vi "ELVIS III v1.0 Read Encoder.vi"(8 "error in (no error)":errorcluster, 9 "Reset Counter":bool, 10 "Channel":T2, 11 "myRIO Ref In":T3) -> (0 "error out":errorcluster, 1 "Counter Direction":T1, 2 "Counter Value":i32, 3 "myRIO Ref Out":T3, 5 "Overflow?":bool)   [LabVIEW 2021]
uses:
  <vilib>/myRIO/Common/Instrument Driver Framework/Utilities/typedefs/myRIO v1.0 Reference.ctl
  <vilib>/myRIO/Common/Instrument Driver Framework/Utilities/typedefs/Generic FPGA Reference.ctl
  <vilib>/myRIO/Common/Instrument Driver Framework/myRIO v1.0/Encoder/typedefs/Encoder Channels Enum.ctl
  <vilib>/myRIO/Common/Instrument Driver Framework/myRIO v1.0/Encoder/typedefs/Encoder Count Direction Enum.ctl
  <vilib>/myRIO/Common/Instrument Driver Framework/ELVIS III v1.0/Encoder/typedefs/ELVIS III Encoder Channels FPGA Reference.ctl
  <vilib>/rvi/errors/niLvFpgaAdjustHostInterfaceError.vi
  <vilib>/rvi/interface/nirviReadWriteControl/nirviReadWriteControl.xnode
  <vilib>/rvi/interface/Simulation/niFpgaSimulationCallBeginRW.vi
  NiFpgaLv.dll
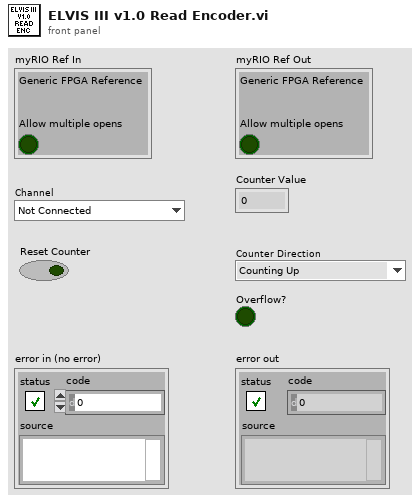
[diagram p1: front panel]
types:
  T1 = typedef "Encoder Count Direction Enum.ctl" = enum16{"Counting Up", "Counting Down"}
  T2 = typedef "Encoder Channels Enum.ctl" = enum16{"Not Connected", "C/ENC0", "C/ENC1", "A/ENC", "A/ENC0", "A/ENC1", "A/ENC2", "A/ENC3", "A/ENC4", "A/ENC5", "A/ENC6", "A/ENC7", "A/ENC8", "A/ENC9", "B/ENC", "B/ENC0", "B/ENC1", "B/ENC2", "B/ENC3", "B/ENC4", "B/ENC5", "B/ENC6", "B/ENC7", "B/ENC8", "B/ENC9", "DIO/ENC0", "DIO/ENC1", "DIO/ENC2", "DIO/ENC3", "DIO/ENC4"}
  T3 = typedef "myRIO v1.0 Reference.ctl" = cluster{"Generic FPGA Reference":T4, "Allow multiple opens":bool}
  T4 = typedef "Generic FPGA Reference.ctl" = refnum<k20>
  T5 = typedef "ELVIS III Encoder Channels FPGA Reference.ctl" = refnum<k20>
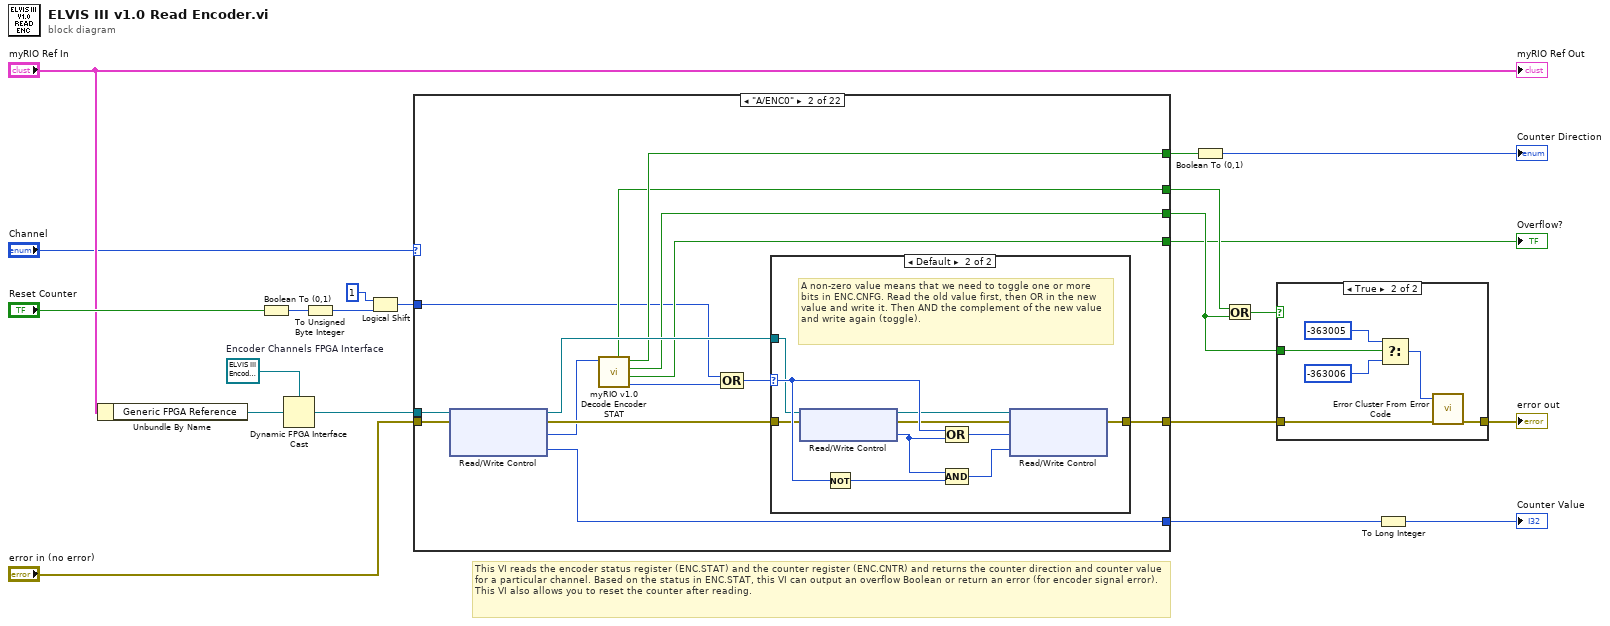
[diagram p0: block diagram]
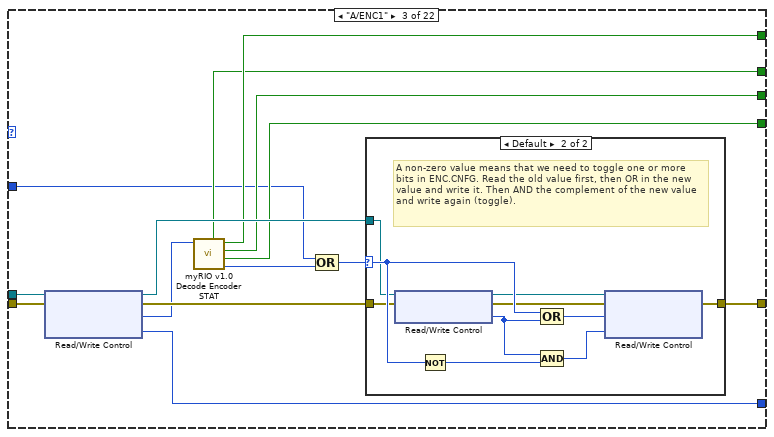
[diagram p4: hidden frame]
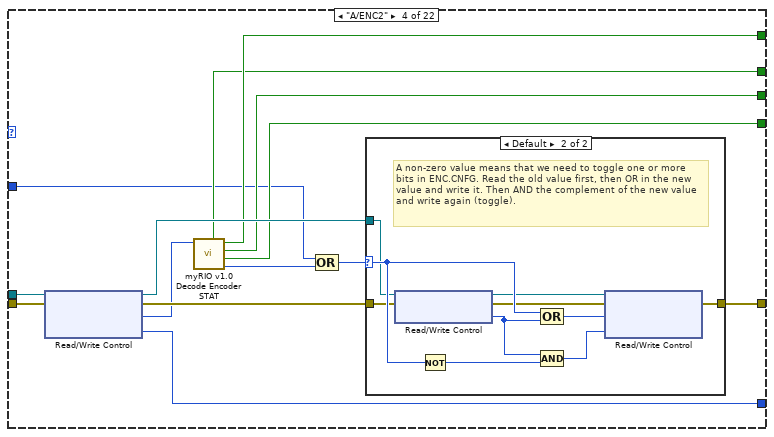
[diagram p6: hidden frame]
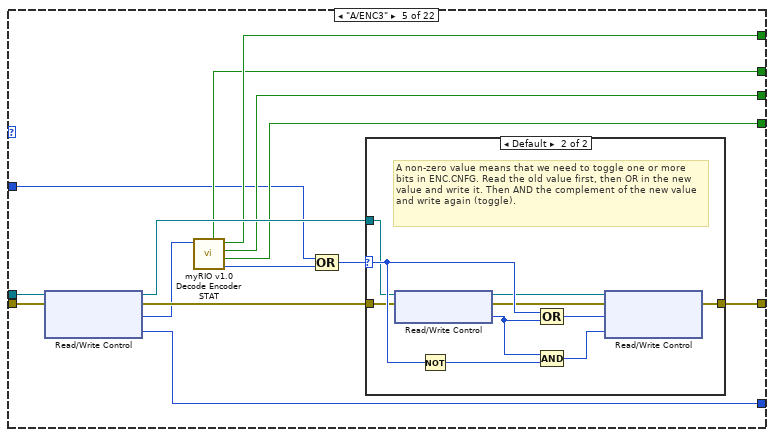
[diagram p8: hidden frame]
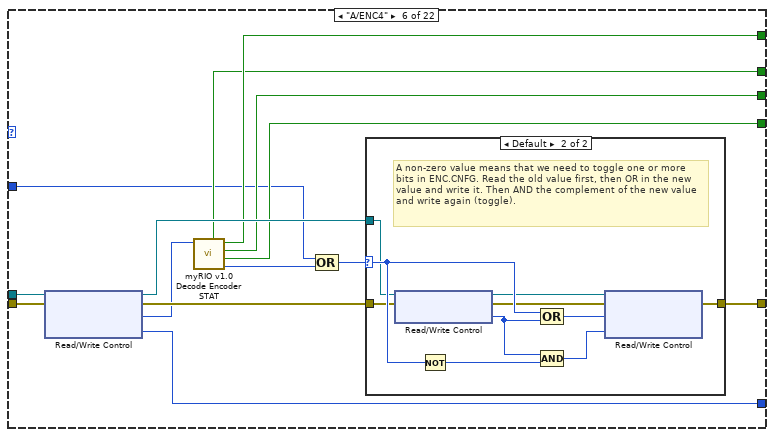
[diagram p10: hidden frame]
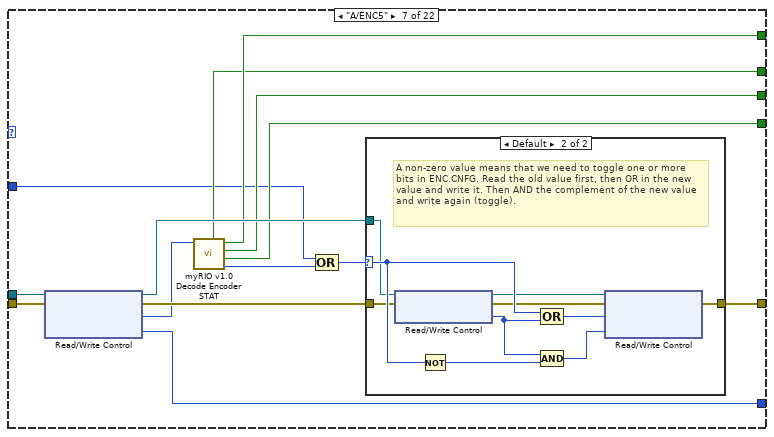
[diagram p12: hidden frame]
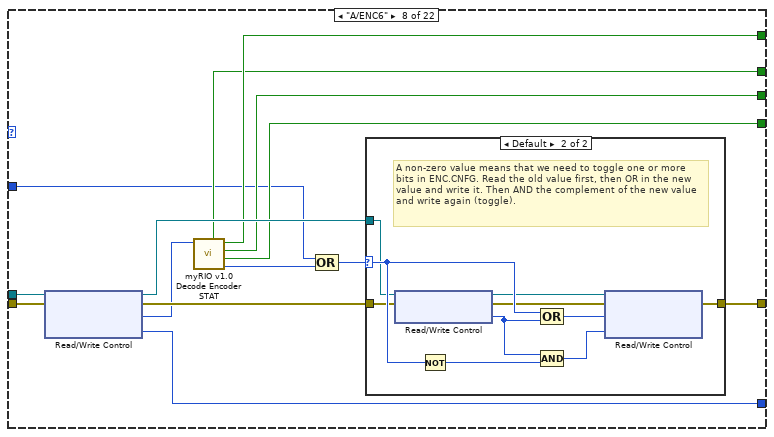
[diagram p14: hidden frame]
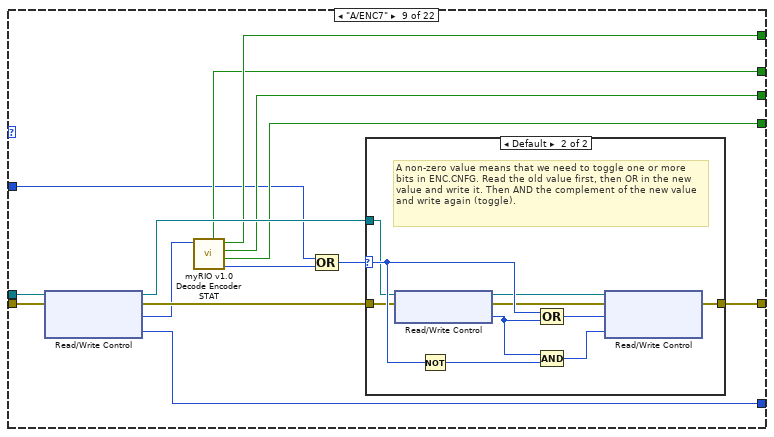
[diagram p16: hidden frame]
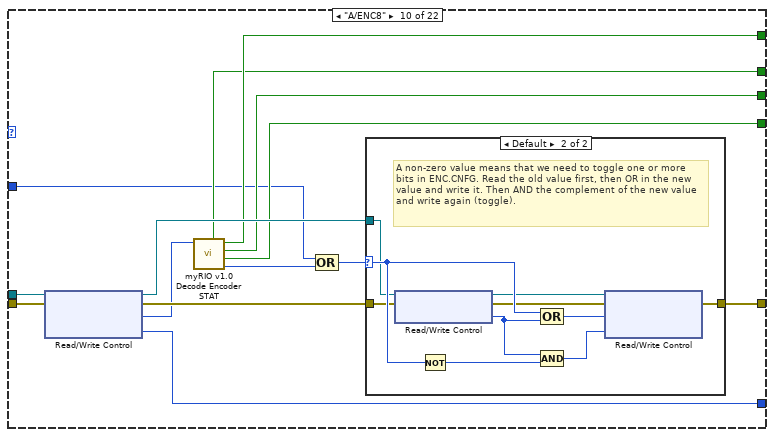
[diagram p18: hidden frame]
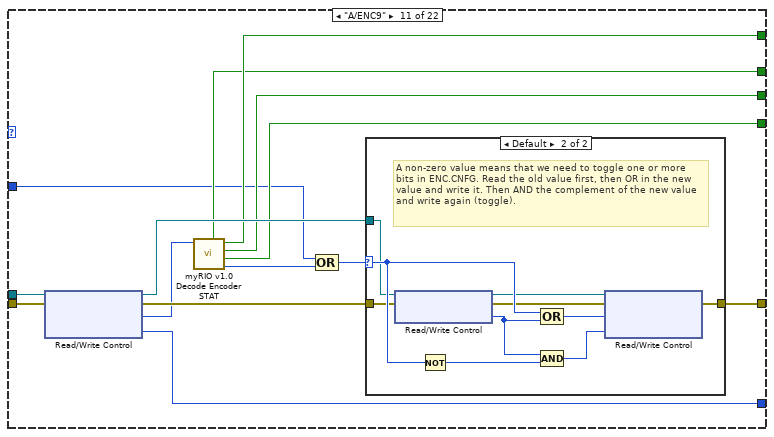
[diagram p20: hidden frame]
diagram:
  w21 = T5 refnum  # Encoder Channels FPGA Interface
  # "This VI reads the encoder status register (ENC.STAT) and the counter register (ENC.CNTR) and returns the counter direction and counter value for a particular channel. Based on the status in ENC.STAT, this VI can output an overflow Boolean or return an error (for encoder signal error). This VI also allows you to reset the counter after reading."
  n1 = Unbundle By Name("myRIO Ref In") -> ("Generic FPGA Reference"=w14:T4)
  n2 = Boolean To (0,1)(Boolean="Reset Counter") -> (0, 1=w15:i16)
  n3 = Dynamic FPGA Interface Cast(Session In=w21, Type=w14) -> (Session Out=w1:T5)
  n4 = To Unsigned Byte Integer(number=w15) -> (unsigned 8bit integer=w16:u8)
  n5 = Logical Shift(y=u8 1, x=w16) -> (x << y=w2:u8)
  n6 = case shown="\"A/ENC0\"" "Channel" {
    tunnel: "error in (no error)" -> [w22 w30 w55 w80 w105 w130 w155 w180 w205 w230 w255 w280 w305 w330 w355 w380 w405 w430 w455 w480 w505 w526]
    tunnel: [w22 w25 w50 w75 w100 w125 w150 w175 w200 w225 w250 w275 w300 w325 w350 w375 w400 w425 w450 w475 w500 w525] -> w9
    tunnel: [_ w24 w49 w74 w99 w124 w149 w174 w199 w224 w249 w274 w299 w324 w349 w374 w399 w424 w449 w474 w499 w524] -> w8
    tunnel: [_ w29 w54 w79 w104 w129 w154 w179 w204 w229 w254 w279 w304 w329 w354 w379 w404 w429 w454 w479 w504 w523] -> w7
    tunnel: [_ w28 w53 w78 w103 w128 w153 w178 w203 w228 w253 w278 w303 w328 w353 w378 w403 w428 w453 w478 w503 w523] -> w6
    tunnel: [_ w27 w52 w77 w102 w127 w152 w177 w202 w227 w252 w277 w302 w327 w352 w377 w402 w427 w452 w477 w502 w523] -> w5
    tunnel: [_ w26 w51 w76 w101 w126 w151 w176 w201 w226 w251 w276 w301 w326 w351 w376 w401 w426 w451 w476 w501 w523] -> w4
    tunnel: w2 -> [_ w23 w48 w73 w98 w123 w148 w173 w198 w223 w248 w273 w298 w323 w348 w373 w398 w423 w448 w473 w498 _]
    tunnel: w1 -> [_ w31 w56 w81 w106 w131 w156 w181 w206 w231 w256 w281 w306 w331 w356 w381 w406 w431 w456 w481 w506 _]
    frame "Not Connected" {
    }
    frame "A/ENC0" {
      n7 = xnode "Read/Write Control"("FPGA VI Reference In"=w31, "error in"=w30) -> ("FPGA VI Reference Out"=w34:T5, "error out"=w33:errorcluster, "ENC.A_0.STAT"=w32:u8, "ENC.A_0.CNTR"=w24:u32)
      n8 = call <vilib>:"myRIO v1.0 Decode Encoder STAT.vi"("ENC.STAT"=w32) -> ("ENC.CNFG to write"=w35:u8, "Signed Overflow?"=w26:bool, "Error?"=w27:bool, "Counting down?"=w29:bool, "Signed Overflow Error?"=w28:bool)  [unwired: 6 in]
      n9 = Compound Arithmetic op=OR(w23, w35) -> (w36:u8)
      n10 = case shown="Default" w36 {
        selector: w36 -> [_ w46]
        tunnel: w34 -> [_ w45]
        tunnel: w33 -> [w37 w44]
        tunnel: [w37 w38] -> w25
        frame 0 {
        }
        frame Default {
          # "A non-zero value means that we need to toggle one or more bits in ENC.CNFG. Read the old value first, then OR in the new value and write it. Then AND the complement of the new value and write again (toggle)."
          n11 = xnode "Read/Write Control"("FPGA VI Reference In"=w45, "error in"=w44) -> ("FPGA VI Reference Out"=w42:T5, "error out"=w41:errorcluster, "ENC.A_0.CNFG"=w43:u8)
          n12 = Not(x=w46) -> (.not. x?=w47:u8)
          n13 = Compound Arithmetic op=OR(w46, w43) -> (w40:u8)
          n14 = Compound Arithmetic op=AND(w43, w47) -> (w39:u8)
          n15 = xnode "Read/Write Control"("FPGA VI Reference In"=w42, "error in"=w41, "ENC.A_0.CNFG"=w40, "ENC.A_0.CNFG"=w39) -> ("error out"=w38:errorcluster)  [unwired: 1 out]
        }
      }
    }
    frame "A/ENC1" {
      n16 = xnode "Read/Write Control"("FPGA VI Reference In"=w56, "error in"=w55) -> ("FPGA VI Reference Out"=w59:T5, "error out"=w58:errorcluster, "ENC.A_1.STAT"=w57:u8, "ENC.A_1.CNTR"=w49:u32)
      n17 = call <vilib>:"myRIO v1.0 Decode Encoder STAT.vi"("ENC.STAT"=w57) -> ("ENC.CNFG to write"=w60:u8, "Signed Overflow?"=w51:bool, "Error?"=w52:bool, "Counting down?"=w54:bool, "Signed Overflow Error?"=w53:bool)  [unwired: 6 in]
      n18 = Compound Arithmetic op=OR(w48, w60) -> (w61:u8)
      n19 = case shown="Default" w61 {
        selector: w61 -> [_ w71]
        tunnel: w59 -> [_ w70]
        tunnel: w58 -> [w62 w69]
        tunnel: [w62 w63] -> w50
        frame 0 {
        }
        frame Default {
          # "A non-zero value means that we need to toggle one or more bits in ENC.CNFG. Read the old value first, then OR in the new value and write it. Then AND the complement of the new value and write again (toggle)."
          n20 = xnode "Read/Write Control"("FPGA VI Reference In"=w70, "error in"=w69) -> ("FPGA VI Reference Out"=w67:T5, "error out"=w66:errorcluster, "ENC.A_1.CNFG"=w68:u8)
          n21 = Not(x=w71) -> (.not. x?=w72:u8)
          n22 = Compound Arithmetic op=OR(w71, w68) -> (w65:u8)
          n23 = Compound Arithmetic op=AND(w68, w72) -> (w64:u8)
          n24 = xnode "Read/Write Control"("FPGA VI Reference In"=w67, "error in"=w66, "ENC.A_1.CNFG"=w65, "ENC.A_1.CNFG"=w64) -> ("error out"=w63:errorcluster)  [unwired: 1 out]
        }
      }
    }
    frame "A/ENC2" {
      n25 = xnode "Read/Write Control"("FPGA VI Reference In"=w81, "error in"=w80) -> ("FPGA VI Reference Out"=w84:T5, "error out"=w83:errorcluster, "ENC.A_2.STAT"=w82:u8, "ENC.A_2.CNTR"=w74:u32)
      n26 = call <vilib>:"myRIO v1.0 Decode Encoder STAT.vi"("ENC.STAT"=w82) -> ("ENC.CNFG to write"=w85:u8, "Signed Overflow?"=w76:bool, "Error?"=w77:bool, "Counting down?"=w79:bool, "Signed Overflow Error?"=w78:bool)  [unwired: 6 in]
      n27 = Compound Arithmetic op=OR(w73, w85) -> (w86:u8)
      n28 = case shown="Default" w86 {
        selector: w86 -> [_ w96]
        tunnel: w84 -> [_ w95]
        tunnel: w83 -> [w87 w94]
        tunnel: [w87 w88] -> w75
        frame 0 {
        }
        frame Default {
          # "A non-zero value means that we need to toggle one or more bits in ENC.CNFG. Read the old value first, then OR in the new value and write it. Then AND the complement of the new value and write again (toggle)."
          n29 = xnode "Read/Write Control"("FPGA VI Reference In"=w95, "error in"=w94) -> ("FPGA VI Reference Out"=w92:T5, "error out"=w91:errorcluster, "ENC.A_2.CNFG"=w93:u8)
          n30 = Not(x=w96) -> (.not. x?=w97:u8)
          n31 = Compound Arithmetic op=OR(w96, w93) -> (w90:u8)
          n32 = Compound Arithmetic op=AND(w93, w97) -> (w89:u8)
          n33 = xnode "Read/Write Control"("FPGA VI Reference In"=w92, "error in"=w91, "ENC.A_2.CNFG"=w90, "ENC.A_2.CNFG"=w89) -> ("error out"=w88:errorcluster)  [unwired: 1 out]
        }
      }
    }
    frame "A/ENC3" {
      n34 = xnode "Read/Write Control"("FPGA VI Reference In"=w106, "error in"=w105) -> ("FPGA VI Reference Out"=w109:T5, "error out"=w108:errorcluster, "ENC.A_3.STAT"=w107:u8, "ENC.A_3.CNTR"=w99:u32)
      n35 = call <vilib>:"myRIO v1.0 Decode Encoder STAT.vi"("ENC.STAT"=w107) -> ("ENC.CNFG to write"=w110:u8, "Signed Overflow?"=w101:bool, "Error?"=w102:bool, "Counting down?"=w104:bool, "Signed Overflow Error?"=w103:bool)  [unwired: 6 in]
      n36 = Compound Arithmetic op=OR(w98, w110) -> (w111:u8)
      n37 = case shown="Default" w111 {
        selector: w111 -> [_ w121]
        tunnel: w109 -> [_ w120]
        tunnel: w108 -> [w112 w119]
        tunnel: [w112 w113] -> w100
        frame 0 {
        }
        frame Default {
          # "A non-zero value means that we need to toggle one or more bits in ENC.CNFG. Read the old value first, then OR in the new value and write it. Then AND the complement of the new value and write again (toggle)."
          n38 = xnode "Read/Write Control"("FPGA VI Reference In"=w120, "error in"=w119) -> ("FPGA VI Reference Out"=w117:T5, "error out"=w116:errorcluster, "ENC.A_3.CNFG"=w118:u8)
          n39 = Not(x=w121) -> (.not. x?=w122:u8)
          n40 = Compound Arithmetic op=OR(w121, w118) -> (w115:u8)
          n41 = Compound Arithmetic op=AND(w118, w122) -> (w114:u8)
          n42 = xnode "Read/Write Control"("FPGA VI Reference In"=w117, "error in"=w116, "ENC.A_3.CNFG"=w115, "ENC.A_3.CNFG"=w114) -> ("error out"=w113:errorcluster)  [unwired: 1 out]
        }
      }
    }
    frame "A/ENC4" {
      n43 = xnode "Read/Write Control"("FPGA VI Reference In"=w131, "error in"=w130) -> ("FPGA VI Reference Out"=w134:T5, "error out"=w133:errorcluster, "ENC.A_4.STAT"=w132:u8, "ENC.A_4.CNTR"=w124:u32)
      n44 = call <vilib>:"myRIO v1.0 Decode Encoder STAT.vi"("ENC.STAT"=w132) -> ("ENC.CNFG to write"=w135:u8, "Signed Overflow?"=w126:bool, "Error?"=w127:bool, "Counting down?"=w129:bool, "Signed Overflow Error?"=w128:bool)  [unwired: 6 in]
      n45 = Compound Arithmetic op=OR(w123, w135) -> (w136:u8)
      n46 = case shown="Default" w136 {
        selector: w136 -> [_ w146]
        tunnel: w134 -> [_ w145]
        tunnel: w133 -> [w137 w144]
        tunnel: [w137 w138] -> w125
        frame 0 {
        }
        frame Default {
          # "A non-zero value means that we need to toggle one or more bits in ENC.CNFG. Read the old value first, then OR in the new value and write it. Then AND the complement of the new value and write again (toggle)."
          n47 = xnode "Read/Write Control"("FPGA VI Reference In"=w145, "error in"=w144) -> ("FPGA VI Reference Out"=w142:T5, "error out"=w141:errorcluster, "ENC.A_4.CNFG"=w143:u8)
          n48 = Not(x=w146) -> (.not. x?=w147:u8)
          n49 = Compound Arithmetic op=OR(w146, w143) -> (w140:u8)
          n50 = Compound Arithmetic op=AND(w143, w147) -> (w139:u8)
          n51 = xnode "Read/Write Control"("FPGA VI Reference In"=w142, "error in"=w141, "ENC.A_4.CNFG"=w140, "ENC.A_4.CNFG"=w139) -> ("error out"=w138:errorcluster)  [unwired: 1 out]
        }
      }
    }
    frame "A/ENC5" {
      n52 = xnode "Read/Write Control"("FPGA VI Reference In"=w156, "error in"=w155) -> ("FPGA VI Reference Out"=w159:T5, "error out"=w158:errorcluster, "ENC.A_5.STAT"=w157:u8, "ENC.A_5.CNTR"=w149:u32)
      n53 = call <vilib>:"myRIO v1.0 Decode Encoder STAT.vi"("ENC.STAT"=w157) -> ("ENC.CNFG to write"=w160:u8, "Signed Overflow?"=w151:bool, "Error?"=w152:bool, "Counting down?"=w154:bool, "Signed Overflow Error?"=w153:bool)  [unwired: 6 in]
      n54 = Compound Arithmetic op=OR(w148, w160) -> (w161:u8)
      n55 = case shown="Default" w161 {
        selector: w161 -> [_ w171]
        tunnel: w159 -> [_ w170]
        tunnel: w158 -> [w162 w169]
        tunnel: [w162 w163] -> w150
        frame 0 {
        }
        frame Default {
          # "A non-zero value means that we need to toggle one or more bits in ENC.CNFG. Read the old value first, then OR in the new value and write it. Then AND the complement of the new value and write again (toggle)."
          n56 = xnode "Read/Write Control"("FPGA VI Reference In"=w170, "error in"=w169) -> ("FPGA VI Reference Out"=w167:T5, "error out"=w166:errorcluster, "ENC.A_5.CNFG"=w168:u8)
          n57 = Not(x=w171) -> (.not. x?=w172:u8)
          n58 = Compound Arithmetic op=OR(w171, w168) -> (w165:u8)
          n59 = Compound Arithmetic op=AND(w168, w172) -> (w164:u8)
          n60 = xnode "Read/Write Control"("FPGA VI Reference In"=w167, "error in"=w166, "ENC.A_5.CNFG"=w165, "ENC.A_5.CNFG"=w164) -> ("error out"=w163:errorcluster)  [unwired: 1 out]
        }
      }
    }
    frame "A/ENC6" {
      n61 = xnode "Read/Write Control"("FPGA VI Reference In"=w181, "error in"=w180) -> ("FPGA VI Reference Out"=w184:T5, "error out"=w183:errorcluster, "ENC.A_6.STAT"=w182:u8, "ENC.A_6.CNTR"=w174:u32)
      n62 = call <vilib>:"myRIO v1.0 Decode Encoder STAT.vi"("ENC.STAT"=w182) -> ("ENC.CNFG to write"=w185:u8, "Signed Overflow?"=w176:bool, "Error?"=w177:bool, "Counting down?"=w179:bool, "Signed Overflow Error?"=w178:bool)  [unwired: 6 in]
      n63 = Compound Arithmetic op=OR(w173, w185) -> (w186:u8)
      n64 = case shown="Default" w186 {
        selector: w186 -> [_ w196]
        tunnel: w184 -> [_ w195]
        tunnel: w183 -> [w187 w194]
        tunnel: [w187 w188] -> w175
        frame 0 {
        }
        frame Default {
          # "A non-zero value means that we need to toggle one or more bits in ENC.CNFG. Read the old value first, then OR in the new value and write it. Then AND the complement of the new value and write again (toggle)."
          n65 = xnode "Read/Write Control"("FPGA VI Reference In"=w195, "error in"=w194) -> ("FPGA VI Reference Out"=w192:T5, "error out"=w191:errorcluster, "ENC.A_6.CNFG"=w193:u8)
          n66 = Not(x=w196) -> (.not. x?=w197:u8)
          n67 = Compound Arithmetic op=OR(w196, w193) -> (w190:u8)
          n68 = Compound Arithmetic op=AND(w193, w197) -> (w189:u8)
          n69 = xnode "Read/Write Control"("FPGA VI Reference In"=w192, "error in"=w191, "ENC.A_6.CNFG"=w190, "ENC.A_6.CNFG"=w189) -> ("error out"=w188:errorcluster)  [unwired: 1 out]
        }
      }
    }
    frame "A/ENC7" {
      n70 = xnode "Read/Write Control"("FPGA VI Reference In"=w206, "error in"=w205) -> ("FPGA VI Reference Out"=w209:T5, "error out"=w208:errorcluster, "ENC.A_7.STAT"=w207:u8, "ENC.A_7.CNTR"=w199:u32)
      n71 = call <vilib>:"myRIO v1.0 Decode Encoder STAT.vi"("ENC.STAT"=w207) -> ("ENC.CNFG to write"=w210:u8, "Signed Overflow?"=w201:bool, "Error?"=w202:bool, "Counting down?"=w204:bool, "Signed Overflow Error?"=w203:bool)  [unwired: 6 in]
      n72 = Compound Arithmetic op=OR(w198, w210) -> (w211:u8)
      n73 = case shown="Default" w211 {
        selector: w211 -> [_ w221]
        tunnel: w209 -> [_ w220]
        tunnel: w208 -> [w212 w219]
        tunnel: [w212 w213] -> w200
        frame 0 {
        }
        frame Default {
          # "A non-zero value means that we need to toggle one or more bits in ENC.CNFG. Read the old value first, then OR in the new value and write it. Then AND the complement of the new value and write again (toggle)."
          n74 = xnode "Read/Write Control"("FPGA VI Reference In"=w220, "error in"=w219) -> ("FPGA VI Reference Out"=w217:T5, "error out"=w216:errorcluster, "ENC.A_7.CNFG"=w218:u8)
          n75 = Not(x=w221) -> (.not. x?=w222:u8)
          n76 = Compound Arithmetic op=OR(w221, w218) -> (w215:u8)
          n77 = Compound Arithmetic op=AND(w218, w222) -> (w214:u8)
          n78 = xnode "Read/Write Control"("FPGA VI Reference In"=w217, "error in"=w216, "ENC.A_7.CNFG"=w215, "ENC.A_7.CNFG"=w214) -> ("error out"=w213:errorcluster)  [unwired: 1 out]
        }
      }
    }
    frame "A/ENC8" {
      n79 = xnode "Read/Write Control"("FPGA VI Reference In"=w231, "error in"=w230) -> ("FPGA VI Reference Out"=w234:T5, "error out"=w233:errorcluster, "ENC.A_8.STAT"=w232:u8, "ENC.A_8.CNTR"=w224:u32)
      n80 = call <vilib>:"myRIO v1.0 Decode Encoder STAT.vi"("ENC.STAT"=w232) -> ("ENC.CNFG to write"=w235:u8, "Signed Overflow?"=w226:bool, "Error?"=w227:bool, "Counting down?"=w229:bool, "Signed Overflow Error?"=w228:bool)  [unwired: 6 in]
      n81 = Compound Arithmetic op=OR(w223, w235) -> (w236:u8)
      n82 = case shown="Default" w236 {
        selector: w236 -> [_ w246]
        tunnel: w234 -> [_ w245]
        tunnel: w233 -> [w237 w244]
        tunnel: [w237 w238] -> w225
        frame 0 {
        }
        frame Default {
          # "A non-zero value means that we need to toggle one or more bits in ENC.CNFG. Read the old value first, then OR in the new value and write it. Then AND the complement of the new value and write again (toggle)."
          n83 = xnode "Read/Write Control"("FPGA VI Reference In"=w245, "error in"=w244) -> ("FPGA VI Reference Out"=w242:T5, "error out"=w241:errorcluster, "ENC.A_8.CNFG"=w243:u8)
          n84 = Not(x=w246) -> (.not. x?=w247:u8)
          n85 = Compound Arithmetic op=OR(w246, w243) -> (w240:u8)
          n86 = Compound Arithmetic op=AND(w243, w247) -> (w239:u8)
          n87 = xnode "Read/Write Control"("FPGA VI Reference In"=w242, "error in"=w241, "ENC.A_8.CNFG"=w240, "ENC.A_8.CNFG"=w239) -> ("error out"=w238:errorcluster)  [unwired: 1 out]
        }
      }
    }
    frame "A/ENC9" {
      n88 = xnode "Read/Write Control"("FPGA VI Reference In"=w256, "error in"=w255) -> ("FPGA VI Reference Out"=w259:T5, "error out"=w258:errorcluster, "ENC.A_9.STAT"=w257:u8, "ENC.A_9.CNTR"=w249:u32)
      n89 = call <vilib>:"myRIO v1.0 Decode Encoder STAT.vi"("ENC.STAT"=w257) -> ("ENC.CNFG to write"=w260:u8, "Signed Overflow?"=w251:bool, "Error?"=w252:bool, "Counting down?"=w254:bool, "Signed Overflow Error?"=w253:bool)  [unwired: 6 in]
      n90 = Compound Arithmetic op=OR(w248, w260) -> (w261:u8)
      n91 = case shown="Default" w261 {
        selector: w261 -> [_ w271]
        tunnel: w259 -> [_ w270]
        tunnel: w258 -> [w262 w269]
        tunnel: [w262 w263] -> w250
        frame 0 {
        }
        frame Default {
          # "A non-zero value means that we need to toggle one or more bits in ENC.CNFG. Read the old value first, then OR in the new value and write it. Then AND the complement of the new value and write again (toggle)."
          n92 = xnode "Read/Write Control"("FPGA VI Reference In"=w270, "error in"=w269) -> ("FPGA VI Reference Out"=w267:T5, "error out"=w266:errorcluster, "ENC.A_9.CNFG"=w268:u8)
          n93 = Not(x=w271) -> (.not. x?=w272:u8)
          n94 = Compound Arithmetic op=OR(w271, w268) -> (w265:u8)
          n95 = Compound Arithmetic op=AND(w268, w272) -> (w264:u8)
          n96 = xnode "Read/Write Control"("FPGA VI Reference In"=w267, "error in"=w266, "ENC.A_9.CNFG"=w265, "ENC.A_9.CNFG"=w264) -> ("error out"=w263:errorcluster)  [unwired: 1 out]
        }
      }
    }
    frame "B/ENC0" {
      n97 = xnode "Read/Write Control"("FPGA VI Reference In"=w281, "error in"=w280) -> ("FPGA VI Reference Out"=w284:T5, "error out"=w283:errorcluster, "ENC.B_0.STAT"=w282:u8, "ENC.B_0.CNTR"=w274:u32)
      n98 = call <vilib>:"myRIO v1.0 Decode Encoder STAT.vi"("ENC.STAT"=w282) -> ("ENC.CNFG to write"=w285:u8, "Signed Overflow?"=w276:bool, "Error?"=w277:bool, "Counting down?"=w279:bool, "Signed Overflow Error?"=w278:bool)  [unwired: 6 in]
      n99 = Compound Arithmetic op=OR(w273, w285) -> (w286:u8)
      n100 = case shown="Default" w286 {
        selector: w286 -> [_ w296]
        tunnel: w284 -> [_ w295]
        tunnel: w283 -> [w287 w294]
        tunnel: [w287 w288] -> w275
        frame 0 {
        }
        frame Default {
          # "A non-zero value means that we need to toggle one or more bits in ENC.CNFG. Read the old value first, then OR in the new value and write it. Then AND the complement of the new value and write again (toggle)."
          n101 = xnode "Read/Write Control"("FPGA VI Reference In"=w295, "error in"=w294) -> ("FPGA VI Reference Out"=w292:T5, "error out"=w291:errorcluster, "ENC.B_0.CNFG"=w293:u8)
          n102 = Not(x=w296) -> (.not. x?=w297:u8)
          n103 = Compound Arithmetic op=OR(w296, w293) -> (w290:u8)
          n104 = Compound Arithmetic op=AND(w293, w297) -> (w289:u8)
          n105 = xnode "Read/Write Control"("FPGA VI Reference In"=w292, "error in"=w291, "ENC.B_0.CNFG"=w290, "ENC.B_0.CNFG"=w289) -> ("error out"=w288:errorcluster)  [unwired: 1 out]
        }
      }
    }
    frame "B/ENC1" {
      n106 = xnode "Read/Write Control"("FPGA VI Reference In"=w306, "error in"=w305) -> ("FPGA VI Reference Out"=w309:T5, "error out"=w308:errorcluster, "ENC.B_1.STAT"=w307:u8, "ENC.B_1.CNTR"=w299:u32)
      n107 = call <vilib>:"myRIO v1.0 Decode Encoder STAT.vi"("ENC.STAT"=w307) -> ("ENC.CNFG to write"=w310:u8, "Signed Overflow?"=w301:bool, "Error?"=w302:bool, "Counting down?"=w304:bool, "Signed Overflow Error?"=w303:bool)  [unwired: 6 in]
      n108 = Compound Arithmetic op=OR(w298, w310) -> (w311:u8)
      n109 = case shown="Default" w311 {
        selector: w311 -> [_ w321]
        tunnel: w309 -> [_ w320]
        tunnel: w308 -> [w312 w319]
        tunnel: [w312 w313] -> w300
        frame 0 {
        }
        frame Default {
          # "A non-zero value means that we need to toggle one or more bits in ENC.CNFG. Read the old value first, then OR in the new value and write it. Then AND the complement of the new value and write again (toggle)."
          n110 = xnode "Read/Write Control"("FPGA VI Reference In"=w320, "error in"=w319) -> ("FPGA VI Reference Out"=w317:T5, "error out"=w316:errorcluster, "ENC.B_1.CNFG"=w318:u8)
          n111 = Not(x=w321) -> (.not. x?=w322:u8)
          n112 = Compound Arithmetic op=OR(w321, w318) -> (w315:u8)
          n113 = Compound Arithmetic op=AND(w318, w322) -> (w314:u8)
          n114 = xnode "Read/Write Control"("FPGA VI Reference In"=w317, "error in"=w316, "ENC.B_1.CNFG"=w315, "ENC.B_1.CNFG"=w314) -> ("error out"=w313:errorcluster)  [unwired: 1 out]
        }
      }
    }
    frame "B/ENC2" {
      n115 = xnode "Read/Write Control"("FPGA VI Reference In"=w331, "error in"=w330) -> ("FPGA VI Reference Out"=w334:T5, "error out"=w333:errorcluster, "ENC.B_2.STAT"=w332:u8, "ENC.B_2.CNTR"=w324:u32)
      n116 = call <vilib>:"myRIO v1.0 Decode Encoder STAT.vi"("ENC.STAT"=w332) -> ("ENC.CNFG to write"=w335:u8, "Signed Overflow?"=w326:bool, "Error?"=w327:bool, "Counting down?"=w329:bool, "Signed Overflow Error?"=w328:bool)  [unwired: 6 in]
      n117 = Compound Arithmetic op=OR(w323, w335) -> (w336:u8)
      n118 = case shown="Default" w336 {
        selector: w336 -> [_ w346]
        tunnel: w334 -> [_ w345]
        tunnel: w333 -> [w337 w344]
        tunnel: [w337 w338] -> w325
        frame 0 {
        }
        frame Default {
          # "A non-zero value means that we need to toggle one or more bits in ENC.CNFG. Read the old value first, then OR in the new value and write it. Then AND the complement of the new value and write again (toggle)."
          n119 = xnode "Read/Write Control"("FPGA VI Reference In"=w345, "error in"=w344) -> ("FPGA VI Reference Out"=w342:T5, "error out"=w341:errorcluster, "ENC.B_2.CNFG"=w343:u8)
          n120 = Not(x=w346) -> (.not. x?=w347:u8)
          n121 = Compound Arithmetic op=OR(w346, w343) -> (w340:u8)
          n122 = Compound Arithmetic op=AND(w343, w347) -> (w339:u8)
          n123 = xnode "Read/Write Control"("FPGA VI Reference In"=w342, "error in"=w341, "ENC.B_2.CNFG"=w340, "ENC.B_2.CNFG"=w339) -> ("error out"=w338:errorcluster)  [unwired: 1 out]
        }
      }
    }
    frame "B/ENC3" {
      n124 = xnode "Read/Write Control"("FPGA VI Reference In"=w356, "error in"=w355) -> ("FPGA VI Reference Out"=w359:T5, "error out"=w358:errorcluster, "ENC.B_3.STAT"=w357:u8, "ENC.B_3.CNTR"=w349:u32)
      n125 = call <vilib>:"myRIO v1.0 Decode Encoder STAT.vi"("ENC.STAT"=w357) -> ("ENC.CNFG to write"=w360:u8, "Signed Overflow?"=w351:bool, "Error?"=w352:bool, "Counting down?"=w354:bool, "Signed Overflow Error?"=w353:bool)  [unwired: 6 in]
      n126 = Compound Arithmetic op=OR(w348, w360) -> (w361:u8)
      n127 = case shown="Default" w361 {
        selector: w361 -> [_ w371]
        tunnel: w359 -> [_ w370]
        tunnel: w358 -> [w362 w369]
        tunnel: [w362 w363] -> w350
        frame 0 {
        }
        frame Default {
          # "A non-zero value means that we need to toggle one or more bits in ENC.CNFG. Read the old value first, then OR in the new value and write it. Then AND the complement of the new value and write again (toggle)."
          n128 = xnode "Read/Write Control"("FPGA VI Reference In"=w370, "error in"=w369) -> ("FPGA VI Reference Out"=w367:T5, "error out"=w366:errorcluster, "ENC.B_3.CNFG"=w368:u8)
          n129 = Not(x=w371) -> (.not. x?=w372:u8)
          n130 = Compound Arithmetic op=OR(w371, w368) -> (w365:u8)
          n131 = Compound Arithmetic op=AND(w368, w372) -> (w364:u8)
          n132 = xnode "Read/Write Control"("FPGA VI Reference In"=w367, "error in"=w366, "ENC.B_3.CNFG"=w365, "ENC.B_3.CNFG"=w364) -> ("error out"=w363:errorcluster)  [unwired: 1 out]
        }
      }
    }
    frame "B/ENC4" {
      n133 = xnode "Read/Write Control"("FPGA VI Reference In"=w381, "error in"=w380) -> ("FPGA VI Reference Out"=w384:T5, "error out"=w383:errorcluster, "ENC.B_4.STAT"=w382:u8, "ENC.B_4.CNTR"=w374:u32)
      n134 = call <vilib>:"myRIO v1.0 Decode Encoder STAT.vi"("ENC.STAT"=w382) -> ("ENC.CNFG to write"=w385:u8, "Signed Overflow?"=w376:bool, "Error?"=w377:bool, "Counting down?"=w379:bool, "Signed Overflow Error?"=w378:bool)  [unwired: 6 in]
      n135 = Compound Arithmetic op=OR(w373, w385) -> (w386:u8)
      n136 = case shown="Default" w386 {
        selector: w386 -> [_ w396]
        tunnel: w384 -> [_ w395]
        tunnel: w383 -> [w387 w394]
        tunnel: [w387 w388] -> w375
        frame 0 {
        }
        frame Default {
          # "A non-zero value means that we need to toggle one or more bits in ENC.CNFG. Read the old value first, then OR in the new value and write it. Then AND the complement of the new value and write again (toggle)."
          n137 = xnode "Read/Write Control"("FPGA VI Reference In"=w395, "error in"=w394) -> ("FPGA VI Reference Out"=w392:T5, "error out"=w391:errorcluster, "ENC.B_4.CNFG"=w393:u8)
          n138 = Not(x=w396) -> (.not. x?=w397:u8)
          n139 = Compound Arithmetic op=OR(w396, w393) -> (w390:u8)
          n140 = Compound Arithmetic op=AND(w393, w397) -> (w389:u8)
          n141 = xnode "Read/Write Control"("FPGA VI Reference In"=w392, "error in"=w391, "ENC.B_4.CNFG"=w390, "ENC.B_4.CNFG"=w389) -> ("error out"=w388:errorcluster)  [unwired: 1 out]
        }
      }
    }
    frame "B/ENC5" {
      n142 = xnode "Read/Write Control"("FPGA VI Reference In"=w406, "error in"=w405) -> ("FPGA VI Reference Out"=w409:T5, "error out"=w408:errorcluster, "ENC.B_5.STAT"=w407:u8, "ENC.B_5.CNTR"=w399:u32)
      n143 = call <vilib>:"myRIO v1.0 Decode Encoder STAT.vi"("ENC.STAT"=w407) -> ("ENC.CNFG to write"=w410:u8, "Signed Overflow?"=w401:bool, "Error?"=w402:bool, "Counting down?"=w404:bool, "Signed Overflow Error?"=w403:bool)  [unwired: 6 in]
      n144 = Compound Arithmetic op=OR(w398, w410) -> (w411:u8)
      n145 = case shown="Default" w411 {
        selector: w411 -> [_ w421]
        tunnel: w409 -> [_ w420]
        tunnel: w408 -> [w412 w419]
        tunnel: [w412 w413] -> w400
        frame 0 {
        }
        frame Default {
          # "A non-zero value means that we need to toggle one or more bits in ENC.CNFG. Read the old value first, then OR in the new value and write it. Then AND the complement of the new value and write again (toggle)."
          n146 = xnode "Read/Write Control"("FPGA VI Reference In"=w420, "error in"=w419) -> ("FPGA VI Reference Out"=w417:T5, "error out"=w416:errorcluster, "ENC.B_5.CNFG"=w418:u8)
          n147 = Not(x=w421) -> (.not. x?=w422:u8)
          n148 = Compound Arithmetic op=OR(w421, w418) -> (w415:u8)
          n149 = Compound Arithmetic op=AND(w418, w422) -> (w414:u8)
          n150 = xnode "Read/Write Control"("FPGA VI Reference In"=w417, "error in"=w416, "ENC.B_5.CNFG"=w415, "ENC.B_5.CNFG"=w414) -> ("error out"=w413:errorcluster)  [unwired: 1 out]
        }
      }
    }
    frame "B/ENC6" {
      n151 = xnode "Read/Write Control"("FPGA VI Reference In"=w431, "error in"=w430) -> ("FPGA VI Reference Out"=w434:T5, "error out"=w433:errorcluster, "ENC.B_6.STAT"=w432:u8, "ENC.B_6.CNTR"=w424:u32)
      n152 = call <vilib>:"myRIO v1.0 Decode Encoder STAT.vi"("ENC.STAT"=w432) -> ("ENC.CNFG to write"=w435:u8, "Signed Overflow?"=w426:bool, "Error?"=w427:bool, "Counting down?"=w429:bool, "Signed Overflow Error?"=w428:bool)  [unwired: 6 in]
      n153 = Compound Arithmetic op=OR(w423, w435) -> (w436:u8)
      n154 = case shown="Default" w436 {
        selector: w436 -> [_ w446]
        tunnel: w434 -> [_ w445]
        tunnel: w433 -> [w437 w444]
        tunnel: [w437 w438] -> w425
        frame 0 {
        }
        frame Default {
          # "A non-zero value means that we need to toggle one or more bits in ENC.CNFG. Read the old value first, then OR in the new value and write it. Then AND the complement of the new value and write again (toggle)."
          n155 = xnode "Read/Write Control"("FPGA VI Reference In"=w445, "error in"=w444) -> ("FPGA VI Reference Out"=w442:T5, "error out"=w441:errorcluster, "ENC.B_6.CNFG"=w443:u8)
          n156 = Not(x=w446) -> (.not. x?=w447:u8)
          n157 = Compound Arithmetic op=OR(w446, w443) -> (w440:u8)
          n158 = Compound Arithmetic op=AND(w443, w447) -> (w439:u8)
          n159 = xnode "Read/Write Control"("FPGA VI Reference In"=w442, "error in"=w441, "ENC.B_6.CNFG"=w440, "ENC.B_6.CNFG"=w439) -> ("error out"=w438:errorcluster)  [unwired: 1 out]
        }
      }
    }
    frame "B/ENC7" {
      n160 = xnode "Read/Write Control"("FPGA VI Reference In"=w456, "error in"=w455) -> ("FPGA VI Reference Out"=w459:T5, "error out"=w458:errorcluster, "ENC.B_7.STAT"=w457:u8, "ENC.B_7.CNTR"=w449:u32)
      n161 = call <vilib>:"myRIO v1.0 Decode Encoder STAT.vi"("ENC.STAT"=w457) -> ("ENC.CNFG to write"=w460:u8, "Signed Overflow?"=w451:bool, "Error?"=w452:bool, "Counting down?"=w454:bool, "Signed Overflow Error?"=w453:bool)  [unwired: 6 in]
      n162 = Compound Arithmetic op=OR(w448, w460) -> (w461:u8)
      n163 = case shown="Default" w461 {
        selector: w461 -> [_ w471]
        tunnel: w459 -> [_ w470]
        tunnel: w458 -> [w462 w469]
        tunnel: [w462 w463] -> w450
        frame 0 {
        }
        frame Default {
          # "A non-zero value means that we need to toggle one or more bits in ENC.CNFG. Read the old value first, then OR in the new value and write it. Then AND the complement of the new value and write again (toggle)."
          n164 = xnode "Read/Write Control"("FPGA VI Reference In"=w470, "error in"=w469) -> ("FPGA VI Reference Out"=w467:T5, "error out"=w466:errorcluster, "ENC.B_7.CNFG"=w468:u8)
          n165 = Not(x=w471) -> (.not. x?=w472:u8)
          n166 = Compound Arithmetic op=OR(w471, w468) -> (w465:u8)
          n167 = Compound Arithmetic op=AND(w468, w472) -> (w464:u8)
          n168 = xnode "Read/Write Control"("FPGA VI Reference In"=w467, "error in"=w466, "ENC.B_7.CNFG"=w465, "ENC.B_7.CNFG"=w464) -> ("error out"=w463:errorcluster)  [unwired: 1 out]
        }
      }
    }
    frame "B/ENC8" {
      n169 = xnode "Read/Write Control"("FPGA VI Reference In"=w481, "error in"=w480) -> ("FPGA VI Reference Out"=w484:T5, "error out"=w483:errorcluster, "ENC.B_8.STAT"=w482:u8, "ENC.B_8.CNTR"=w474:u32)
      n170 = call <vilib>:"myRIO v1.0 Decode Encoder STAT.vi"("ENC.STAT"=w482) -> ("ENC.CNFG to write"=w485:u8, "Signed Overflow?"=w476:bool, "Error?"=w477:bool, "Counting down?"=w479:bool, "Signed Overflow Error?"=w478:bool)  [unwired: 6 in]
      n171 = Compound Arithmetic op=OR(w473, w485) -> (w486:u8)
      n172 = case shown="Default" w486 {
        selector: w486 -> [_ w496]
        tunnel: w484 -> [_ w495]
        tunnel: w483 -> [w487 w494]
        tunnel: [w487 w488] -> w475
        frame 0 {
        }
        frame Default {
          # "A non-zero value means that we need to toggle one or more bits in ENC.CNFG. Read the old value first, then OR in the new value and write it. Then AND the complement of the new value and write again (toggle)."
          n173 = xnode "Read/Write Control"("FPGA VI Reference In"=w495, "error in"=w494) -> ("FPGA VI Reference Out"=w492:T5, "error out"=w491:errorcluster, "ENC.B_8.CNFG"=w493:u8)
          n174 = Not(x=w496) -> (.not. x?=w497:u8)
          n175 = Compound Arithmetic op=OR(w496, w493) -> (w490:u8)
          n176 = Compound Arithmetic op=AND(w493, w497) -> (w489:u8)
          n177 = xnode "Read/Write Control"("FPGA VI Reference In"=w492, "error in"=w491, "ENC.B_8.CNFG"=w490, "ENC.B_8.CNFG"=w489) -> ("error out"=w488:errorcluster)  [unwired: 1 out]
        }
      }
    }
    frame "B/ENC9" {
      n178 = xnode "Read/Write Control"("FPGA VI Reference In"=w506, "error in"=w505) -> ("FPGA VI Reference Out"=w509:T5, "error out"=w508:errorcluster, "ENC.B_9.STAT"=w507:u8, "ENC.B_9.CNTR"=w499:u32)
      n179 = call <vilib>:"myRIO v1.0 Decode Encoder STAT.vi"("ENC.STAT"=w507) -> ("ENC.CNFG to write"=w510:u8, "Signed Overflow?"=w501:bool, "Error?"=w502:bool, "Counting down?"=w504:bool, "Signed Overflow Error?"=w503:bool)  [unwired: 6 in]
      n180 = Compound Arithmetic op=OR(w498, w510) -> (w511:u8)
      n181 = case shown="Default" w511 {
        selector: w511 -> [_ w521]
        tunnel: w509 -> [_ w520]
        tunnel: w508 -> [w512 w519]
        tunnel: [w512 w513] -> w500
        frame 0 {
        }
        frame Default {
          # "A non-zero value means that we need to toggle one or more bits in ENC.CNFG. Read the old value first, then OR in the new value and write it. Then AND the complement of the new value and write again (toggle)."
          n182 = xnode "Read/Write Control"("FPGA VI Reference In"=w520, "error in"=w519) -> ("FPGA VI Reference Out"=w517:T5, "error out"=w516:errorcluster, "ENC.B_9.CNFG"=w518:u8)
          n183 = Not(x=w521) -> (.not. x?=w522:u8)
          n184 = Compound Arithmetic op=OR(w521, w518) -> (w515:u8)
          n185 = Compound Arithmetic op=AND(w518, w522) -> (w514:u8)
          n186 = xnode "Read/Write Control"("FPGA VI Reference In"=w517, "error in"=w516, "ENC.B_9.CNFG"=w515, "ENC.B_9.CNFG"=w514) -> ("error out"=w513:errorcluster)  [unwired: 1 out]
        }
      }
    }
    frame Default {
      w523 = FALSE ("Counting down?")
      w524 = enum16{""}.""  # Place holder
      # "The channel requested is not supported. This happens when the channel name is valid (a valid channel enum) but there it is not handled in the case structure."
      n187 = call <vilib>:"Error Cluster From Error Code.vi"("error in (no error)"=w526, "error code (0)"=-363003) -> ("error out"=w525:errorcluster)  [unwired: 7 in]
    }
  }
  "Overflow?" <- w4
  n188 = Boolean To (0,1)(Boolean=w7) -> (0, 1=→"Counter Direction":i16)
  n189 = Or(x=w6, y=w5) -> (x .or. y?=w11:bool)
  n190 = case shown="True" w11 {
    tunnel: w9 -> [w528 w533]
    tunnel: [w528 w534] -> w20
    tunnel: w5 -> [_ w532]
    frame False {
    }
    frame True {
      n191 = Select(t=-363005 ("error code (0)"), s=w532, f=-363006 ("error code (0)")) -> (s? t:f=w530:i32)
      n192 = call <vilib>:"Error Cluster From Error Code.vi"("error in (no error)"=w533, "error code (0)"=w530) -> ("error out"=w534:errorcluster)  [unwired: 7 in]
    }
  }
  "error out" <- w20
  n193 = To Long Integer(number=w8) -> (32bit integer=→"Counter Value":i32)
  "myRIO Ref Out" <- "myRIO Ref In"
